vi "GetArrayOfPoints.vi"(11 "file path (dialog if empty)":path=path "/home/lvuser/mp3.csv") -> (1 "Number of Points":i32, 2 "Array of Trajectory Points":dbl[][](array[numeric]))   [LabVIEW 2017]
uses:
  <vilib>/Utility/file.llb/Read Delimited Spreadsheet (DBL).vi
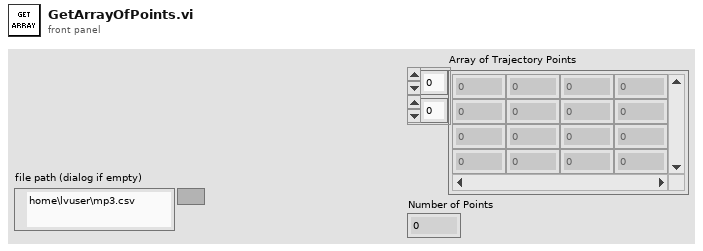
[diagram p1: front panel]
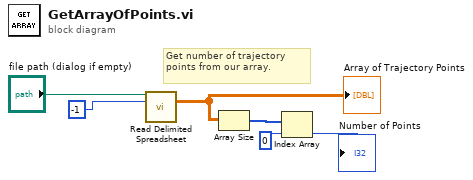
[diagram p0: block diagram]
diagram:
  # "Get number of trajectory points from our array."
  n1 = call-poly <vilib>:"Read Delimited Spreadsheet.vi"("file path (dialog if empty)"="file path (dialog if empty)", "number of rows (all:-1)"=-1) -> ("all rows"=w3:dbl[][])  [unwired: 8 in, 5 out]
  "Array of Trajectory Points" <- w3
  n2 = Array Size(array=w3) -> (size(s)=w4:i32[])
  n3 = Index Array(array=w4, index=0) -> (element=→"Number of Points":i32)
